vi "Call Subpanel VI.vi"(8 "error in (no error)":errorcluster, 10 "VI Refnum":refnum<vi>, 11 "VacuumLine Configuration in":refnum<class "VacuumLine Configuration.lvclass">) -> (0 "error out":errorcluster, 3 "VacuumLine Configuration out":refnum<class "VacuumLine Configuration.lvclass">)   [LabVIEW 2016, in "Hardware.lvlib" / "VacuumLine.lvlib" / "VacuumLine Configuration.lvclass"]
uses:
  <userlib>/Common Components/Hardware/Abstract System/VacuumLine/VacuumLine Config/VacuumLine Configuration.lvclass
  <userlib>/Configuration Dialog Actor/Configuration.lvclass
  C:/Program Files (x86)/National Instruments/LabVIEW 2016/user.lib/Configuration Dialog Actor/Configuration.lvclass
  <userlib>/Configuration Dialog Actor/Configuration.lvclass/Configuration.ctl
  <userlib>/Common Components/Hardware/Motor/Motor Config/Motor Configuration.lvclass
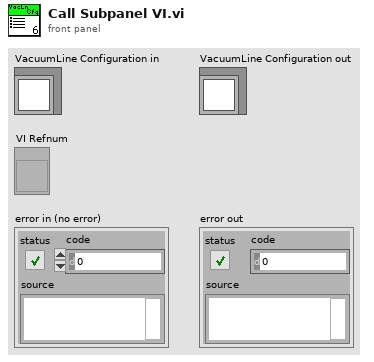
[diagram p1: front panel]
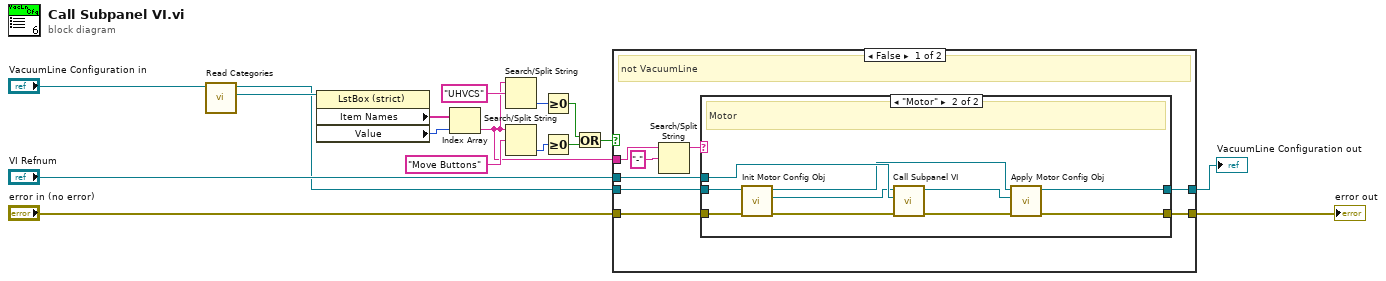
[diagram p0: block diagram]
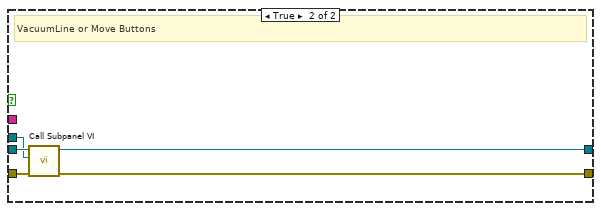
[diagram p3: hidden frame]
diagram:
  n1 = call <userlib>:"Read Categories.vi"("Configuration in"="VacuumLine Configuration in") -> ("Categories"=w17:refnum<vi>, "Configuration out"=w7:refnum<class "VacuumLine Configuration.lvclass">)  [unwired: 8 in, 1 out]
  n2 = property class="LstBox (strict)"(reference=w17) -> ("Item Names"=w16:string[], "Value"=w15:i32)  [unwired: 1 in, 2 out]
  n3 = Index Array(array=w16, index=w15) -> (element=w3:string)
  n4 = Search/Split String(string=w3, search string/char (-)="UHVCS") -> (offset of match=w6:i32)  [unwired: 1 in, 2 out]
  n5 = Search/Split String(string=w3, search string/char (-)="Move Buttons") -> (offset of match=w4:i32)  [unwired: 1 in, 2 out]
  n6 = Greater Or Equal To 0?(x=w6) -> (x >= 0?=w8:bool)
  n7 = Greater Or Equal To 0?(x=w4) -> (x >= 0?=w1:bool)
  n8 = Or(x=w8, y=w1) -> (x .or. y?=w2:bool)
  n9 = case shown="False" w2 {
    tunnel: w7 -> [w25 w42]
    tunnel: "VI Refnum" -> [w24 w38]
    tunnel: "error in (no error)" -> [w23 w41]
    tunnel: [w22 w40] -> w11
    tunnel: [w21 w39] -> w10
    tunnel: w3 -> [w19 _]
    frame False {
      # "not VacuumLine"
      n10 = Search/Split String(string=w19, search string/char (-)="-") -> (substring before match=w18:string)  [unwired: 1 in, 2 out]
      n11 = case shown="\"Motor\"" w18 {
        tunnel: [w26 w32] -> w21
        tunnel: [w27 w31] -> w22
        tunnel: w23 -> [w26 w37]
        tunnel: w24 -> [_ w36]
        tunnel: w25 -> [w27 w33]
        frame Default {
        }
        frame "Motor" {
          # "Motor"
          n12 = call <userlib>:"Init Motor Config Obj.vi"("error in (no error)"=w37, "VacuumLine Configuration in"=w33) -> ("error out"=w34:errorcluster, "Motor Config Obj"=w30:refnum<class "Motor Configuration.lvclass">, "VacuumLine Configuration out"=w29:refnum<class "VacuumLine Configuration.lvclass">)  [unwired: 7 in]
          n13 = call-dynamic "Call Subpanel VI.vi"("error in (no error)"=w34, "VI Refnum"=w36, "Motor Configuration in"=w30) -> ("error out"=w35:errorcluster, "Motor Configuration out"=w28:refnum<class "Motor Configuration.lvclass">)  [unwired: 7 in]
          n14 = call <userlib>:"Apply Motor Config Obj.vi"("error in (no error)"=w35, "Motor Config Obj"=w28, "VacuumLine Configuration in"=w29) -> ("error out"=w32:errorcluster, "VacuumLine Configuration out"=w31:refnum<class "VacuumLine Configuration.lvclass">)  [unwired: 7 in]
        }
      }
    }
    frame True {
      # "VacuumLine or Move Buttons"
      n15 = call-parent "Call Subpanel VI.vi"("error in (no error)"=w41, "VI Refnum"=w38, "Configuration in"=w42) -> ("error out"=w39:errorcluster, "Configuration out"=w40:refnum<class "VacuumLine Configuration.lvclass">)  [unwired: 7 in]
    }
  }
  "error out" <- w10
  "VacuumLine Configuration out" <- w11
